vi "Update Pump State.vi"(8 "error in (no error)":cluster{"状态":bool, "代码":i32, "源":string} caption="错误输入（无错误）", 10 "泵状态":bool, 11 "冷却器UI输入":refnum<class "Live User Controller.lvclass">) -> (0 "error out":cluster{"状态":bool, "代码":i32, "源":string} caption="错误输出", 3 "冷却器UI输出":refnum<class "Live User Controller.lvclass">)   [LabVIEW 2013, in "Live User Controller.lvclass"]
doc: "更新用户接口，显示泵状态。"
uses:
  Live User Controller.lvclass
  Live User Controller.lvclass/Live User Controller.ctl
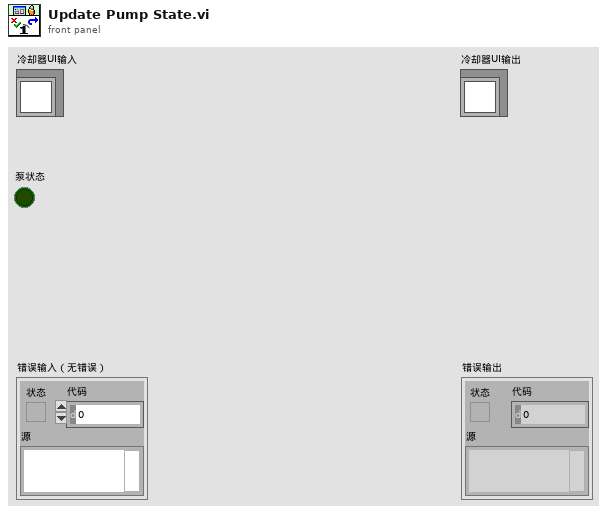
[diagram p1: front panel]
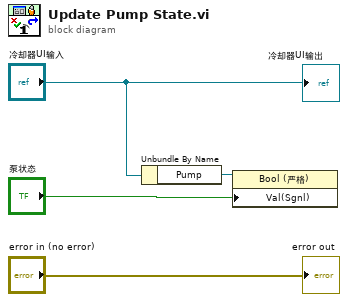
[diagram p0: block diagram]
diagram:
  n1 = Unbundle By Name("冷却器UI输入") -> ("Pump"=w3:refnum<vi>)
  n2 = property class="Bool (严格)"(reference=w3, "Val(Sgnl)"="泵状态") -> ()  [unwired: 1 in, 2 out]
  "error out" <- "error in (no error)"
  "冷却器UI输出" <- "冷却器UI输入"
